vi "test begin.vi"() -> ()   [LabVIEW 2012, in "LightPipes.lvlib"]
uses:
  LightPipes.lvlib
panel:
  in  "Path in":string="C:\\Users\\Green Beret\\Documents\\Visual Studio 2012\\Projects\\LightPipes\\LightPipes\\lp12src\\LabView\\images\\original\\target_intensity.gpl"
  out "field out":T1
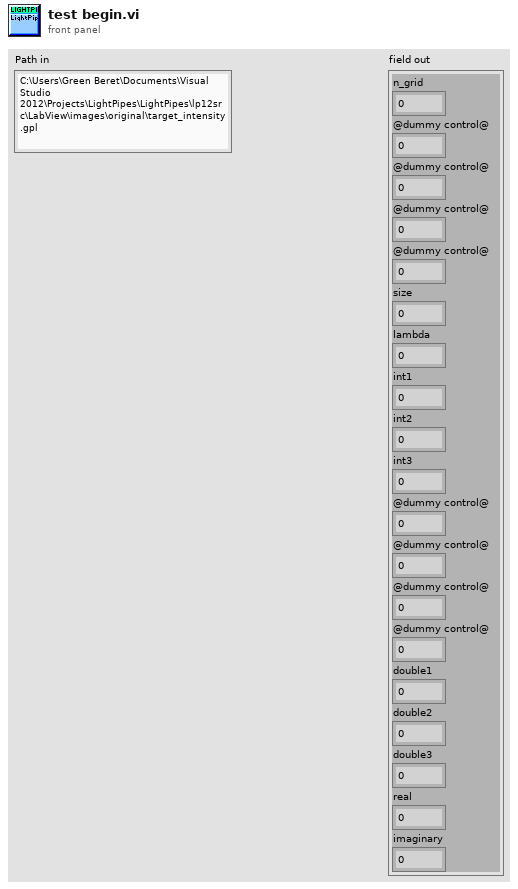
[diagram p1: front panel]
types:
  T1 = cluster{"n_grid":i32, "@dummy control@":i8, "@dummy control@":i8, "@dummy control@":i8, "@dummy control@":i8, "size":dbl, "lambda":dbl, "int1":i32, "int2":i32, "int3":i32, "@dummy control@":i8, "@dummy control@":i8, "@dummy control@":i8, "@dummy control@":i8, "double1":dbl, "double2":dbl, "double3":dbl, "real":u32, "imaginary":u32}
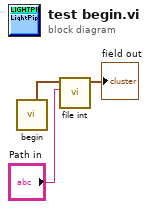
[diagram p0: block diagram]
diagram:
  n1 = call "begin.vi"() -> ("field out"=w2:T1)  [unwired: 11 in]
  n2 = call "file int.vi"("Path in"="Path in", "field"=w2) -> ("field out"=→"field out":T1)  [unwired: 9 in]
